vi "NI PXI Programmable Power Supply Main Page.vi"(8 "error in (no error)":errorcluster, 11 "Node Ptr":T2 format="%.0x") -> (0 "error out":errorcluster)   [LabVIEW 2018, in "NI PXI-4110 Programmable Power Supply Custom Device.lvlib"]
uses:
  NI PXI-4110 Programmable Power Supply Custom Device.lvlib
  <vilib>/NI Veristand/Custom Device API/Custom Device Item Ref.ctl
  Power_Supply_In_Use.ctl
  4110_Global.vi
  <vilib>/NI Veristand/Custom Device API/Get Item Property (String).vi
  <vilib>/NI Veristand/Custom Device API/Get Item Property (U16).vi
  <vilib>/NI Veristand/Custom Device API/Set Item Property (Boolean).vi
  <vilib>/NI Veristand/Custom Device API/Get Item Property (Boolean).vi
  <vilib>/NI Veristand/Custom Device API/Set Item Property (String).vi
  <vilib>/NI Veristand/Custom Device API/Set Item Property (U16).vi
  <vilib>/NI VeriStand/Custom Device API/Custom Device API.lvlib
panel:
  in  "Power Supply In Use":T1
  in  "Power Source":bool
  in  "Power Supply NI-MAX Device Name":string
  in  "Header":cluster{"Section Name":string}={"Section Name"="PXI-4110  Settings"}
  in  "Description":string
  in  "Custom Device Name":string
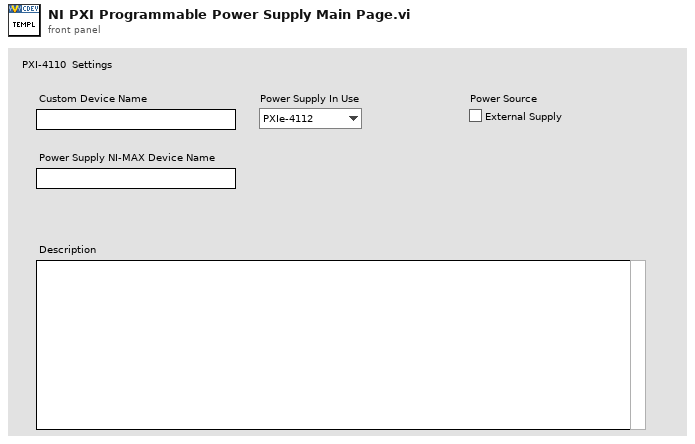
[diagram p1: front panel]
types:
  T1 = typedef "NI PXI-4110 Programmable Power Supply Custom Device.lvlib/Power_Supply_In_Use.ctl" = enum16{"PXIe-4112", "PXI-4110"}
  T2 = typedef "Custom Device API.lvlib/Custom Device Item Ref.ctl" = u64
  T3 = enum8{"Enabled", "Disabled", "Disabled and Grayed Out"}
  T4 = typedef "Custom Device API.lvlib/Custom Device Item Info.ctl" = cluster{"Name":string, "Is Channel":bool, "GUID":string, "Is Waveform":bool}
  T5 = typedef "Custom Device API.lvlib/Custom Device Commands.ctl" = enum16{"Default", "Item renamed", "Shutdown", "Dynamic button pressed"}
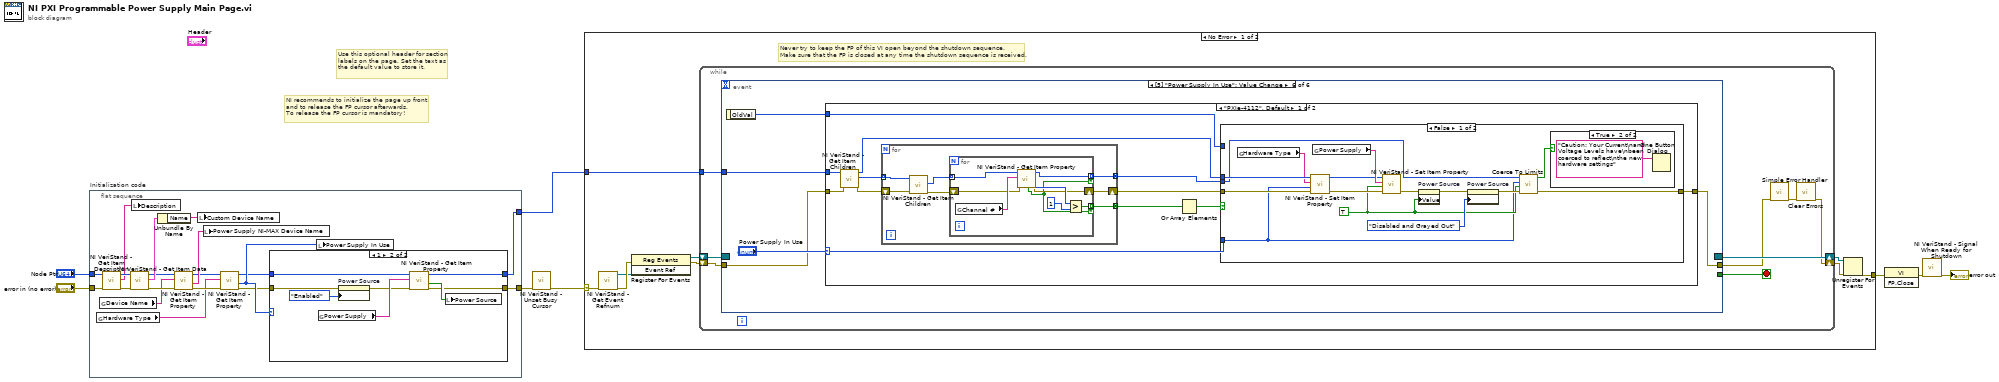
[diagram p0: block diagram]
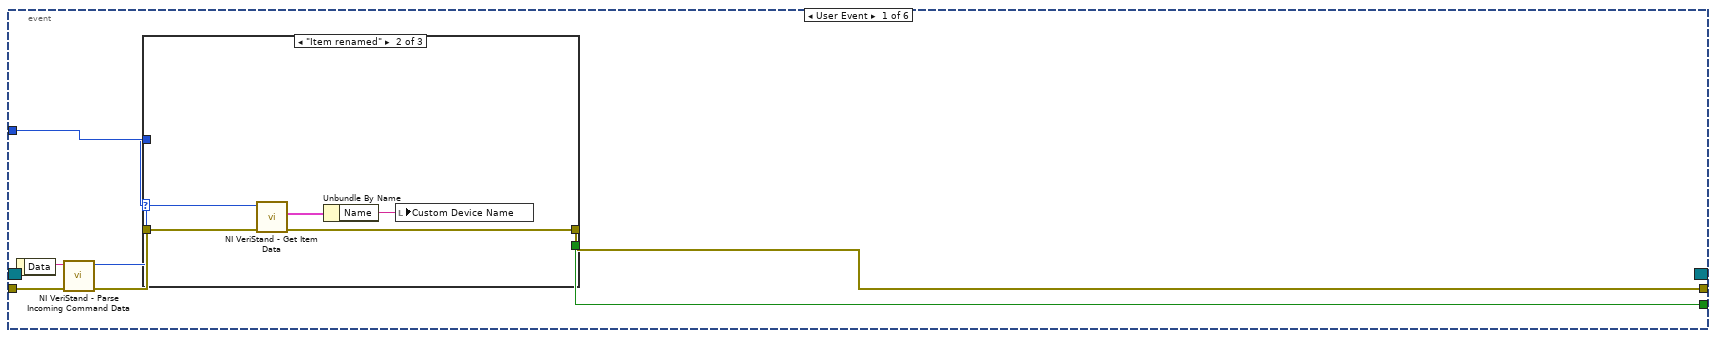
[diagram p2: hidden frame]
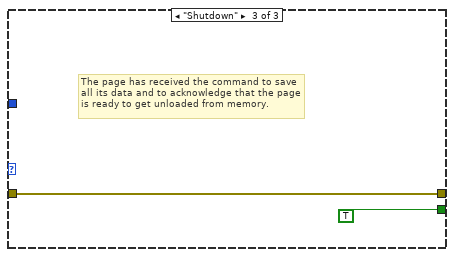
[diagram p4: hidden frame]
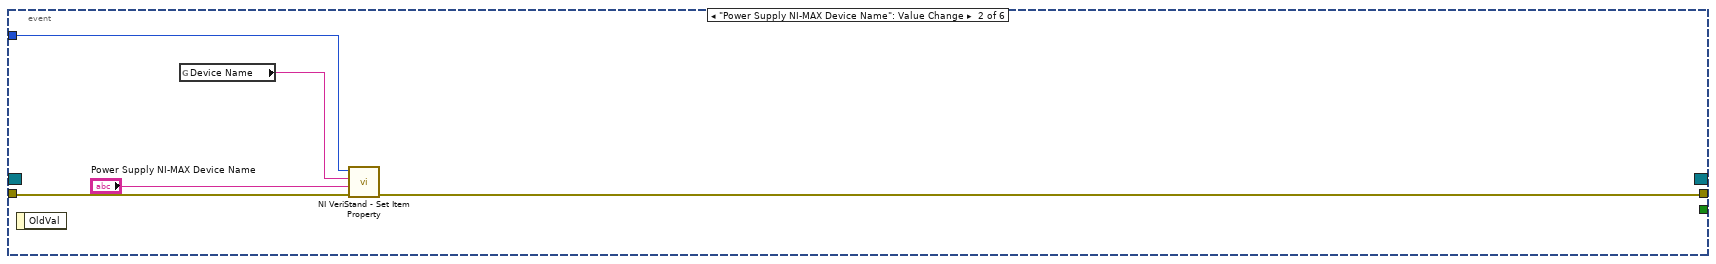
[diagram p5: hidden frame]
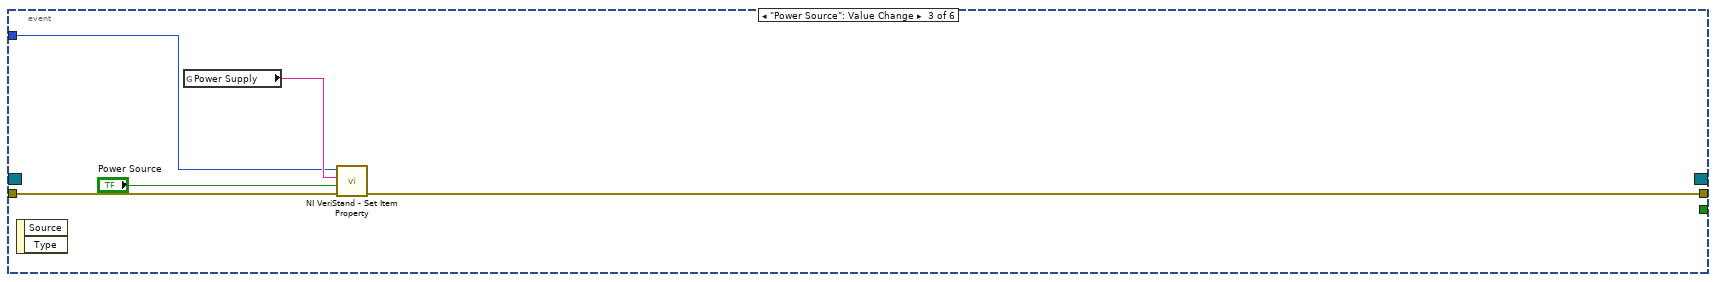
[diagram p6: hidden frame]
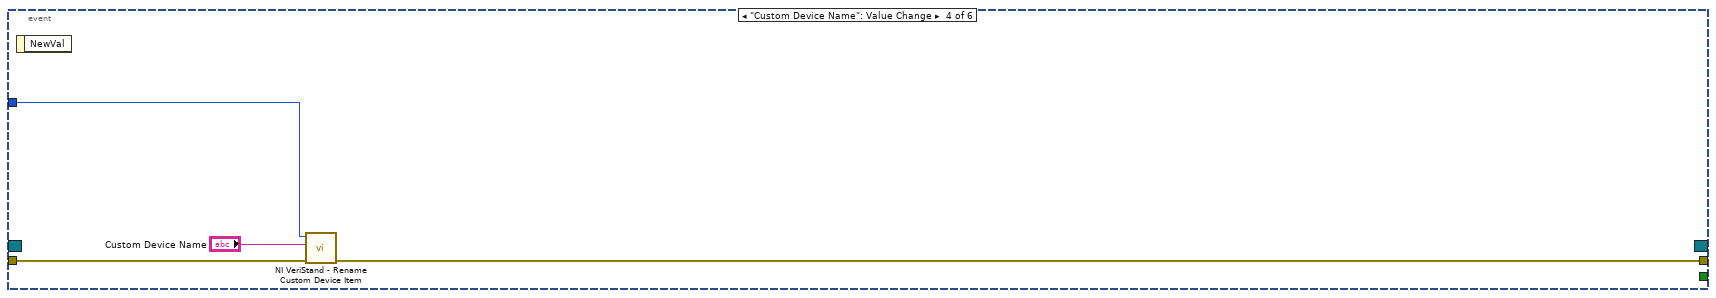
[diagram p7: hidden frame]
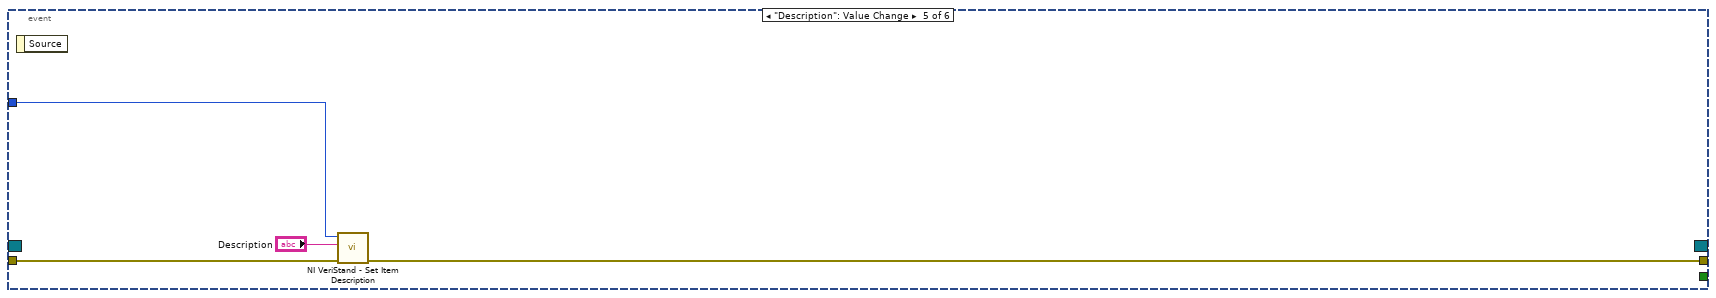
[diagram p8: hidden frame]
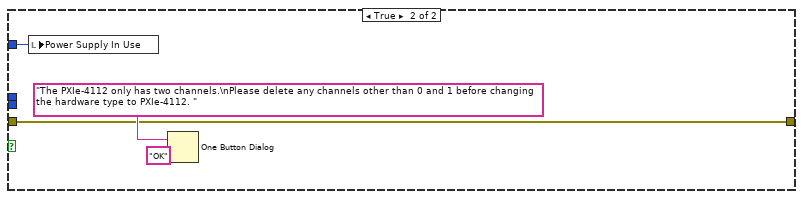
[diagram p10: hidden frame]
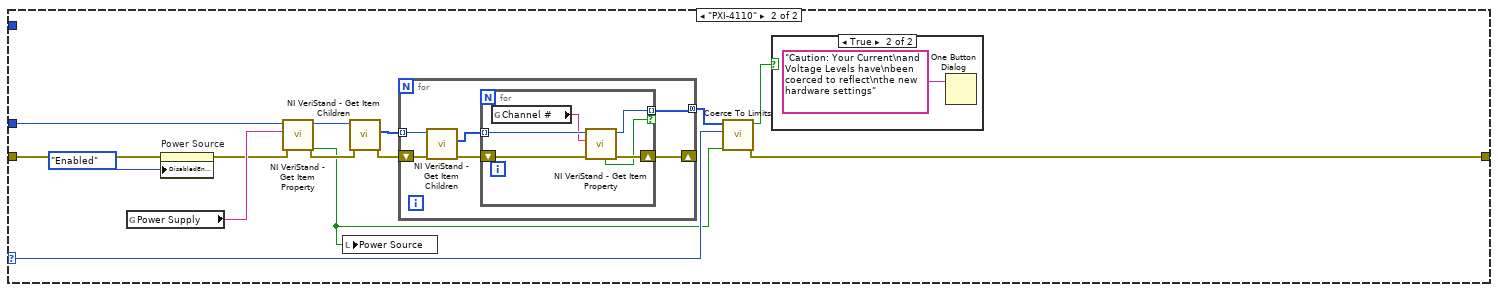
[diagram p11: hidden frame]
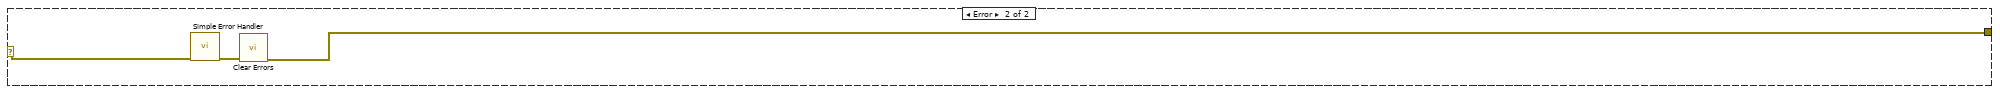
[diagram p13: hidden frame]
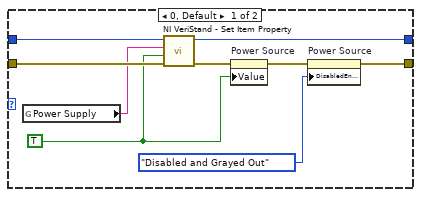
[diagram p14: hidden frame]
diagram:
  # "Use this optional header for section labels on the page. Set the text as the default value to store it."
  # "NI recommends to initialize the page up front\nand to release the FP cursor afterwards.\nTo release the FP cursor is mandatory!"
  n1 = flat-sequence "Initialization code" {
    tunnel: "error in (no error)" -> [w21]
    tunnel: "Node Ptr" -> [w22]
    tunnel: [w9] -> w4
    tunnel: [w11] -> w1
    frame #0 {
      n2 = global read "4110_Global.vi" "Hardware Type"() -> (w14:string)
      n3 = global read "4110_Global.vi" "Device Name"() -> (w18:string)
      n4 = call <vilib>:"NI VeriStand - Get Item Description.vi"("error in (no error)"=w21, "Item Ref in"=w22) -> ("error out"=w25:errorcluster, "Description"=w26:string, "Item Ref out"=w27:T2)  [unwired: 7 out]
      n5 = call <vilib>:"NI VeriStand - Get Item Data.vi"("error in (no error)"=w25, "Item Ref in"=w27) -> ("error out"=w20:errorcluster, "Item Info"=w24:T4, "Item Ref out"=w19:T2)  [unwired: 7 out]
      n6 = local write "Description"(w26) -> ()
      n7 = Unbundle By Name(w24) -> ("Name"=w23:string)
      n8 = call-poly <vilib>:"NI VeriStand - Get Item Property.vi"("error in (no error)"=w20, "Property Name"=w18, "Item Ref in"=w19) -> ("error out"=w15:errorcluster, "Value"=w17:string, "Item Ref out"=w16:T2)  [unwired: 5 in, 1 out]
      n9 = local write "Custom Device Name"(w23) -> ()
      n10 = local write "Power Supply NI-MAX Device Name"(w17) -> ()
      n11 = call-poly <vilib>:"NI VeriStand - Get Item Property.vi"("error in (no error)"=w15, "Property Name"=w14, "Item Ref in"=w16) -> ("error out"=w10:errorcluster, "Value"=w13:u16, "Item Ref out"=w12:T2)  [unwired: 5 in, 1 out]
      n12 = case shown="1" w13 {
        tunnel: [w28 w44] -> w11
        tunnel: w12 -> [w33 w41]
        tunnel: w10 -> [w32 w39]
        tunnel: [w36 w40] -> w9
        frame 0, Default {
          w30 = TRUE ("Power Source")
          n13 = global read "4110_Global.vi" "Power Supply"() -> (w31:string)
          n14 = call-poly <vilib>:"NI VeriStand - Set Item Property.vi"("error in (no error)"=w32, "Value"=w30, "Property Name"=w31, "Item Ref in"=w33) -> ("error out"=w29:errorcluster, "Item Ref out"=w28:T2)  [unwired: 5 in, 1 out]
          n15 = property on="Power Source" class="Bool (strict)"(error in=w29, "Value"=w30) -> (error out=w34:errorcluster)  [unwired: 1 in, 1 out]
          n16 = property on="Power Source" class="Bool (strict)"(error in=w34, "DisabledEnum"=T3."Disabled and Grayed Out" ("Disabled")) -> (error out=w36:errorcluster)  [unwired: 1 in, 1 out]
        }
        frame 1 {
          n17 = global read "4110_Global.vi" "Power Supply"() -> (w43:string)
          n18 = property on="Power Source" class="Bool (strict)"(error in=w39, "DisabledEnum"=T3."Enabled" ("Disabled")) -> (error out=w38:errorcluster)  [unwired: 1 in, 1 out]
          n19 = call-poly <vilib>:"NI VeriStand - Get Item Property.vi"("error in (no error)"=w38, "Property Name"=w43, "Item Ref in"=w41) -> ("error out"=w40:errorcluster, "Value"=w42:bool, "Item Ref out"=w44:T2)  [unwired: 5 in, 1 out]
          n20 = local write "Power Source"(w42) -> ()
        }
      }
      n21 = local write "Power Supply In Use"(w13) -> ()
    }
  }
  n22 = call <vilib>:"NI VeriStand - Unset Busy Cursor.vi"("error in (no error)"=w4) -> ("error out"=w3:errorcluster)  [unwired: 10 out]
  n23 = case shown="No Error" w3 {
    selector: w3 -> [w45 w177]
    tunnel: [w50 w175] -> w8
    tunnel: w1 -> [w46 _]
    frame No Error {
      # "Never try to keep the FP of this VI open beyond the shutdown sequence.\nMake sure that the FP is closed at any time the shutdown sequence is received."
      n24 = call <vilib>:"NI VeriStand - Get Event Refnum.vi"("error in (no error)"=w45) -> ("error out"=w53:errorcluster, "Event Ref"=w49:refnum<user-event>)  [unwired: 9 out]
      n25 = register-events(error in=w53, w49) -> (reference out=w47:refnum<event-registration>, error out=w48:errorcluster)  [unwired: 1 in]
      n26 = while {
        tunnel: w46 -> [w57]
        shift-right: [w54] -> w51
        shift-left: w48 -> [w60]
        shift-right: [w61] -> w52
        shift-left: w47 -> [w59]
        stop <- w58 stop-if-true
        n27 = event shown="[5] \"Power Supply In Use\": Value Change" {
          selector: w59 -> [_ _ _ _ _ _]
          dyn-events: [_ _ _ _ _ _] -> w61
          timeout: _ -> [_ _ _ _ _ _]
          tunnel: w60 -> [w68 w81 w83 w90 w93 w97]
          tunnel: [w64 _ _ _ _ _] -> w58
          tunnel: [w63 w77 w82 w89 w92 w99] -> w56
          tunnel: w57 -> [w62 w80 w85 w88 w94 w96]
          event User Event {
            n28 = event-data() -> ("Data"=w67:string)  [unwired: 1 out]
            n29 = call <vilib>:"NI VeriStand - Parse Incoming Command Data.vi"("error in (no error)"=w68, "Incoming data"=w67) -> ("error out"=w66:errorcluster, "Action"=w65:T5)  [unwired: 8 out]
            n30 = case shown="\"Item renamed\"" w65 {
              tunnel: w66 -> [w69 w74 w75]
              tunnel: [_ _ TRUE] -> w64
              tunnel: [w69 w71 w75] -> w63
              tunnel: w62 -> [_ w73 _]
              frame "Default", Default {
              }
              frame "Item renamed" {
                n31 = call <vilib>:"NI VeriStand - Get Item Data.vi"("error in (no error)"=w74, "Item Ref in"=w73) -> ("error out"=w71:errorcluster, "Item Info"=w72:T4)  [unwired: 8 out]
                n32 = Unbundle By Name(w72) -> ("Name"=w70:string)
                n33 = local write "Custom Device Name"(w70) -> ()
              }
              frame "Shutdown" {
                # "The page has received the command to save all its data and to acknowledge that the page is ready to get unloaded from memory."
              }
            }
          }
          event "Power Supply NI-MAX Device Name": Value Change {
            n34 = event-data() -> ()  [unwired: 2 out]
            n35 = global read "4110_Global.vi" "Device Name"() -> (w79:string)
            n36 = call-poly <vilib>:"NI VeriStand - Set Item Property.vi"("error in (no error)"=w81, "Value"="Power Supply NI-MAX Device Name", "Property Name"=w79, "Item Ref in"=w80) -> ("error out"=w77:errorcluster)  [unwired: 5 in, 2 out]
          }
          event "Power Source": Value Change {
            n37 = event-data() -> ()  [unwired: 3 out]
            n38 = global read "4110_Global.vi" "Power Supply"() -> (w86:string)
            n39 = call-poly <vilib>:"NI VeriStand - Set Item Property.vi"("error in (no error)"=w83, "Value"="Power Source", "Property Name"=w86, "Item Ref in"=w85) -> ("error out"=w82:errorcluster)  [unwired: 5 in, 2 out]
          }
          event "Custom Device Name": Value Change {
            n40 = event-data() -> ()  [unwired: 2 out]
            n41 = call <vilib>:"NI VeriStand - Rename Custom Device Item.vi"("error in (no error)"=w90, "New Name"="Custom Device Name", "Item Ref in"=w88) -> ("error out"=w89:errorcluster)  [unwired: 1 in, 7 out]
          }
          event "Description": Value Change {
            n42 = event-data() -> ()  [unwired: 2 out]
            n43 = call <vilib>:"NI VeriStand - Set Item Description.vi"("error in (no error)"=w93, "Description"="Description", "Item Ref in"=w94) -> ("error out"=w92:errorcluster)  [unwired: 8 out]
          }
          event Value Change {
            n44 = event-data() -> ("OldVal"=w95:T1)  [unwired: 1 out]
            n45 = case shown="\"PXIe-4112\", Default" "Power Supply In Use" {
              selector: "Power Supply In Use" -> [w102 w156]
              tunnel: w96 -> [w109 w160]
              tunnel: w97 -> [w108 w159]
              tunnel: [w101 w151] -> w99
              tunnel: w95 -> [w105 _]
              frame "PXIe-4112", Default {
                n46 = call <vilib>:"NI VeriStand - Get Item Children.vi"("error in (no error)"=w108, "Item Ref in"=w109) -> ("error out"=w110:errorcluster, "Child Refs"=w111:T2[], "Item Ref out"=w104:T2)  [unwired: 6 in, 1 out]
                n47 = for {
                  tunnel: w111 -> [w114] mode=indexing
                  tunnel: [w118] -> w107 mode=concatenating
                  tunnel: [w116] -> w100 mode=concatenating
                  shift-right: [w117] -> w103
                  shift-left: w110 -> [w115]
                  n48 = call <vilib>:"NI VeriStand - Get Item Children.vi"("error in (no error)"=w115, "Item Ref in"=w114) -> ("error out"=w113:errorcluster, "Child Refs"=w112:T2[])  [unwired: 6 in, 2 out]
                  n49 = for {
                    tunnel: w112 -> [w127] mode=indexing
                    tunnel: [w122] -> w118 mode=indexing if=w119
                    shift-right: [w121] -> w117
                    shift-left: w113 -> [w125]
                    tunnel: [w120] -> w116 mode=indexing if=w119
                    n50 = global read "4110_Global.vi" "Channel #"() -> (w126:string)
                    n51 = call-poly <vilib>:"NI VeriStand - Get Item Property.vi"("error in (no error)"=w125, "Property Name"=w126, "Item Ref in"=w127) -> ("error out"=w121:errorcluster, "Value"=w124:u16, "Item Ref out"=w120:T2, "Found?"=w119:bool)  [unwired: 5 in]
                    n52 = Greater?(x=w124, y=u16 1) -> (0:w122:bool)
                  }
                }
                n53 = Or Array Elements(Boolean array=w107) -> (logical OR=w106:bool)
                n54 = case shown="False" w106 {
                  tunnel: w105 -> [_ w145]
                  tunnel: w104 -> [w138 _]
                  tunnel: w103 -> [w137 w144]
                  tunnel: w102 -> [w129 _]
                  tunnel: [w132 w144] -> w101
                  tunnel: w100 -> [w131 _]
                  frame False {
                    w130 = TRUE ("Power Source")
                    n55 = global read "4110_Global.vi" "Hardware Type"() -> (w136:string)
                    n56 = call-poly <vilib>:"NI VeriStand - Set Item Property.vi"("error in (no error)"=w137, "Value"=w129, "Property Name"=w136, "Item Ref in"=w138) -> ("error out"=w134:errorcluster, "Item Ref out"=w135:T2)  [unwired: 5 in, 1 out]
                    n57 = global read "4110_Global.vi" "Power Supply"() -> (w141:string)
                    n58 = call-poly <vilib>:"NI VeriStand - Set Item Property.vi"("error in (no error)"=w134, "Value"=w130, "Property Name"=w141, "Item Ref in"=w135) -> ("error out"=w140:errorcluster)  [unwired: 5 in, 2 out]
                    n59 = property on="Power Source" class="Bool (strict)"(error in=w140, "Value"=w130) -> (error out=w142:errorcluster)  [unwired: 1 in, 1 out]
                    n60 = property on="Power Source" class="Bool (strict)"(error in=w142, "DisabledEnum"=T3."Disabled and Grayed Out" ("Disabled")) -> (error out=w133:errorcluster)  [unwired: 1 in, 1 out]
                    n61 = call "Coerce To Limits.vi"("error in (no error)"=w133, "External Supply?"=w130, "Power Supply In Use"=w129, "Channels to Coerce"=w131) -> ("error out"=w132:errorcluster, "Values Coerced?"=w128:bool)  [unwired: 6 in]
                    n62 = case shown="True" w128 {
                      frame False {
                      }
                      frame True {
                        n63 = One Button Dialog(message="Caution: Your Current\nand Voltage Levels have\nbeen coerced to reflect\nthe new hardware settings") -> ()  [unwired: 1 in, 1 out]
                      }
                    }
                  }
                  frame True {
                    n64 = local write "Power Supply In Use"(w145) -> ()
                    n65 = One Button Dialog(message="The PXIe-4112 only has two channels.\nPlease delete any channels other than 0 and 1 before changing the hardware type to PXIe-4112. ", button name ("OK")="OK") -> ()  [unwired: 1 out]
                  }
                }
              }
              frame "PXI-4110" {
                n66 = global read "4110_Global.vi" "Power Supply"() -> (w161:string)
                n67 = property on="Power Source" class="Bool (strict)"(error in=w159, "DisabledEnum"=T3."Enabled" ("Disabled")) -> (error out=w158:errorcluster)  [unwired: 1 in, 1 out]
                n68 = call-poly <vilib>:"NI VeriStand - Get Item Property.vi"("error in (no error)"=w158, "Property Name"=w161, "Item Ref in"=w160) -> ("error out"=w155:errorcluster, "Value"=w153:bool, "Item Ref out"=w154:T2)  [unwired: 5 in, 1 out]
                n69 = local write "Power Source"(w153) -> ()
                n70 = call <vilib>:"NI VeriStand - Get Item Children.vi"("error in (no error)"=w155, "Item Ref in"=w154) -> ("error out"=w149:errorcluster, "Child Refs"=w150:T2[])  [unwired: 6 in, 2 out]
                n71 = for {
                  tunnel: w150 -> [w167] mode=indexing
                  shift-right: [w163] -> _
                  shift-left: w149 -> [w166]
                  tunnel: [w162] -> w148 mode=concatenating
                  n72 = call <vilib>:"NI VeriStand - Get Item Children.vi"("error in (no error)"=w166, "Item Ref in"=w167) -> ("error out"=w164:errorcluster, "Child Refs"=w165:T2[])  [unwired: 6 in, 2 out]
                  n73 = for {
                    tunnel: w165 -> [w173] mode=indexing
                    shift-right: [w170] -> w163
                    shift-left: w164 -> [w171]
                    tunnel: [w169] -> w162 mode=indexing if=w168
                    n74 = global read "4110_Global.vi" "Channel #"() -> (w172:string)
                    n75 = call-poly <vilib>:"NI VeriStand - Get Item Property.vi"("error in (no error)"=w171, "Property Name"=w172, "Item Ref in"=w173) -> ("error out"=w170:errorcluster, "Item Ref out"=w169:T2, "Found?"=w168:bool)  [unwired: 5 in, 1 out]
                  }
                }
                n76 = call "Coerce To Limits.vi"("External Supply?"=w153, "Power Supply In Use"=w156, "Channels to Coerce"=w148) -> ("error out"=w151:errorcluster, "Values Coerced?"=w152:bool)  [unwired: 7 in]
                n77 = case shown="True" w152 {
                  frame False {
                  }
                  frame True {
                    n78 = One Button Dialog(message="Caution: Your Current\nand Voltage Levels have\nbeen coerced to reflect\nthe new hardware settings") -> ()  [unwired: 1 in, 1 out]
                  }
                }
              }
            }
          }
        }
        n79 = call <vilib>:"Simple Error Handler.vi"("error in (no error)"=w56) -> ("error out"=w55:errorcluster)  [unwired: 1 in, 7 out]
        n80 = call <vilib>:"Clear Errors.vi"("error in (no error)"=w55) -> ("error out"=w54:errorcluster)  [unwired: 1 in, 5 out]
      }
      n81 = Unregister For Events(event registration refnum=w52, error in=w51) -> (error out=w50:errorcluster)
    }
    frame Error {
      n82 = call <vilib>:"Simple Error Handler.vi"("error in (no error)"=w177) -> ("error out"=w176:errorcluster)  [unwired: 1 in, 7 out]
      n83 = call <vilib>:"Clear Errors.vi"("error in (no error)"=w176) -> ("error out"=w175:errorcluster)  [unwired: 1 in, 5 out]
    }
  }
  n84 = invoke class="VI" method="FP.Close"(error in=w8) -> (error out=w7:errorcluster)  [unwired: 2 in, 2 out]
  n85 = call <vilib>:"NI VeriStand - Signal When Ready for Shutdown.vi"("error in (no error)"=w7) -> ("error out"=→"error out":errorcluster)  [unwired: 10 out]
